vi "Threshold Img v2.vi"(8 "error in (no error)":errorcluster, 9 "Threshold":sgl=128.0 format="%.2f", 10 "Img Dst":T1, 11 "Img Src":T1) -> (0 "error out":errorcluster, 3 "Thresh Img":T1)   [LabVIEW 2013]
uses:
  <vilib>/vision/Image Controls.llb/IMAQ Image.ctl
  <vilib>/vision/NI_Vision_Development_Module.lvlib
panel:
  out "Img Threshold":T1(plugin-control)
  out "Img src":T1(plugin-control)
  in  "Upper limit":sgl=256.0 format="%.2f"
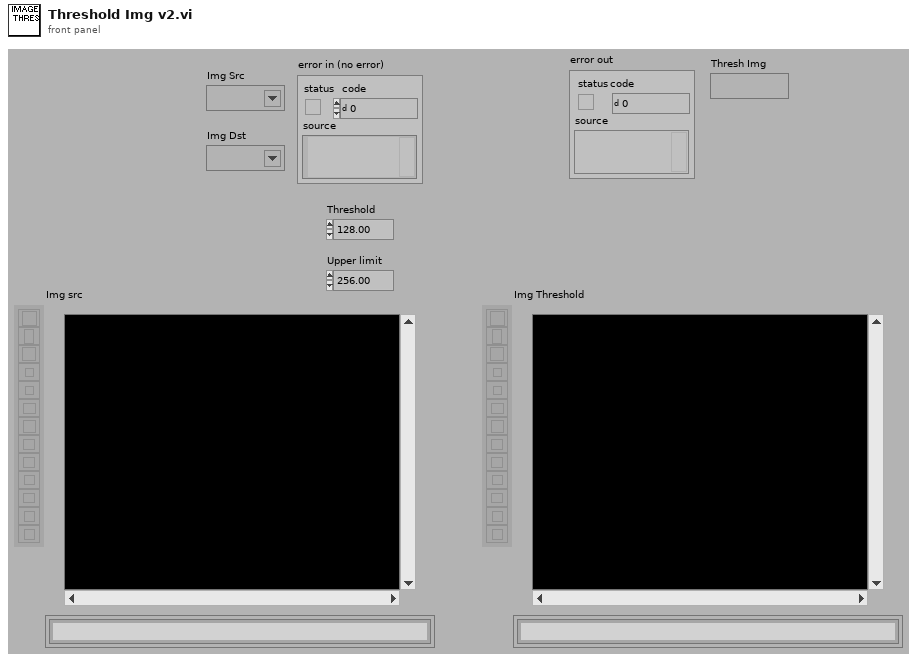
[diagram p1: front panel]
types:
  T1 = typedef "IMAQ Image.ctl" = refnum<image>
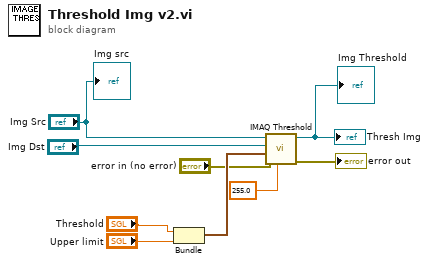
[diagram p0: block diagram]
diagram:
  n1 = Bundle("Threshold"="Threshold", "Upper limit"="Upper limit") -> (w5:cluster{"Threshold":sgl, "Upper limit":sgl})  [unwired: 1 out]
  n2 = call "IMAQ Threshold"("Replace Value"=sgl 255.0, "error in (no error)"="error in (no error)", "Range"=w5, "Image Dst"="Img Dst", "Image Src"="Img Src") -> ("error out"=→"error out":errorcluster, "Image Dst Out"=→"Thresh Img" →"Img Threshold":T1)  [unwired: 1 in, 4 out]
  "Img src" <- "Img Src"
